vi "get status.vi"(8 "error in (no error)":errorcluster, 11 "channel":u16 format="%x") -> (0 "error out":errorcluster, 3 "status":u32 format="%x")   [LabVIEW 2024, in "atsj peakcan basic.lvlib"]
doc: "Gets the current bus status of a PeakCAN <b>channel</b>."
uses:
  atsj peakcan basic.lvlib
  support/x64/PCANBasic.dll
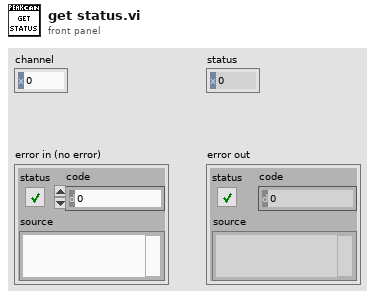
[diagram p1: front panel]
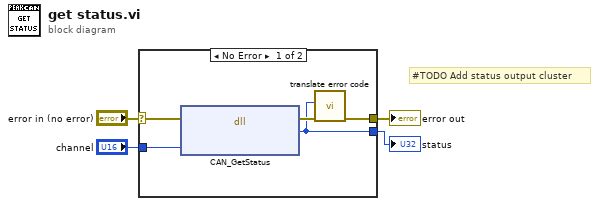
[diagram p0: block diagram]
diagram:
  # "#TODO Add status output cluster"
  n1 = case shown="No Error" "error in (no error)" {
    selector: "error in (no error)" -> [w8 w10]
    tunnel: [w6 w10] -> w3
    tunnel: "channel" -> [w9 _]
    tunnel: [w5 _] -> w1
    frame No Error {
      n2 = dll-call lib="C:/atsj/plateau/atsj-peakcan-basic-for-labview/src/support/x64/PCANBasic.dll" fn="CAN_GetStatus" ("get status")(error in=w8, "Channel"=w9) -> (error out=w7:errorcluster, "Status"=w5:u32)  [unwired: 3 in, 1 out]
      n3 = call "translate error code.vi"("error in (no error)"=w7, "error code"=w5) -> ("error out"=w6:errorcluster)  [unwired: 9 in]
    }
    frame Error {
    }
  }
  "error out" <- w3
  "status" <- w1
